vi "DIO_ReadAll.vi"(7 "Device Index":i32 max=32, 8 "error in (no error)":errorcluster) -> (0 "error out":errorcluster, 2 "Boolean array":bool[][](array[boolean]), 3 "Output":u8[](array[numeric]))   [LabVIEW 2012]
doc: "This VI can be used to read all the bits an an ACCES USB-DIO board."
uses:
  Windows/System32/AIOUSB.dll
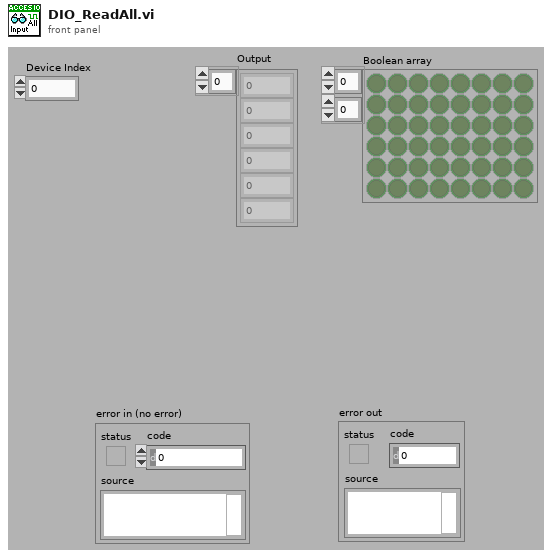
[diagram p1: front panel]
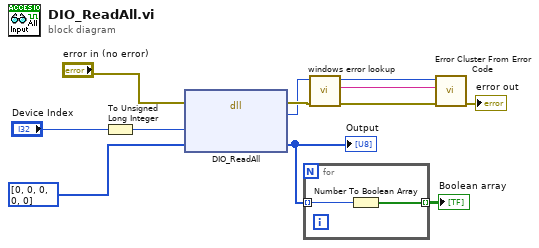
[diagram p0: block diagram]
diagram:
  n1 = To Unsigned Long Integer(number="Device Index") -> (unsigned 32bit integer=w1:u32)
  n2 = dll-call lib="C:/Windows/System32/AIOUSB.dll" fn="DIO_ReadAll"(error in="error in (no error)", "DeviceIndex"=w1, "Buffer"=u8[] [0, 0, 0, 0, 0] ("Array")) -> (error out=w4:errorcluster, w3:u32, "Buffer"=w9:u8[])  [unwired: 3 in, 1 out]
  "Output" <- w9
  n3 = for {
    tunnel: w9 -> [w13] mode=indexing
    tunnel: [w12] -> w8 mode=indexing
    n4 = Number To Boolean Array(number=w13) -> (Boolean array=w12:bool[])
  }
  "Boolean array" <- w8
  n5 = call "windows error lookup.vi"("error in (no error)"=w4, "Error Code"=w3) -> ("error out"=w5:errorcluster, "error message (\"\")"=w7:string)  [unwired: 8 in]
  n6 = call <vilib>:"Error Cluster From Error Code.vi"("error in (no error)"=w5, "error message (\"\")"=w7, "error code (0)"=w3) -> ("error out"=→"error out":errorcluster)  [unwired: 6 in]
